vi "Insert Item(s).vi"   [LabVIEW 2017, in "JSONtext.lvlib"]
doc: "Insert item(s) into a JSON Object."
uses:
  JSONtext.lvlib
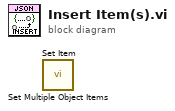
[diagram p0: block diagram]
diagram:
  n1 = call "Set Multiple Object Items.vi"() -> ()  [unwired: 9 in, 2 out]
  n2 = call "Set Item.vi"() -> ()  [unwired: 8 in, 3 out]
